vi "Close virtual shutter.vi"(8 "Error In":errorcluster) -> (0 "error out":errorcluster)   [LabVIEW 2020]
uses:
  Typedefs/Shutter state.ctl
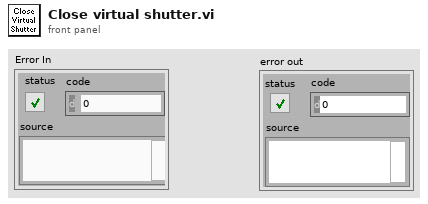
[diagram p1: front panel]
types:
  T1 = typedef "Shutter state.ctl" = enum16{"Closed/Disabled", "Open/Enabled"}
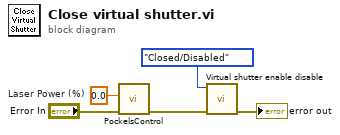
[diagram p0: block diagram]
diagram:
  w4 = 0.0  # Laser Power (%)
  n1 = call "PockelsControl.vi"("Error In"="Error In", "Laser Power (%)"=w4) -> ("Error Out"=w2:errorcluster)  [unwired: 9 in]
  n2 = call "Virtual shutter enable disable.vi"("error in (no error)"=w2, "Virtual Shutter"=Shutter_state."Closed/Disabled") -> ("error out"=→"error out":errorcluster)  [unwired: 9 in]
